vi "Align Window on Parent.vi"(8 "error in (no error)":errorcluster, 10 "Parent VI":refnum<vi>, 11 "VI in":refnum<vi>) -> (0 "error out":errorcluster, 3 "VI out":refnum<vi>)   [LabVIEW 2020]
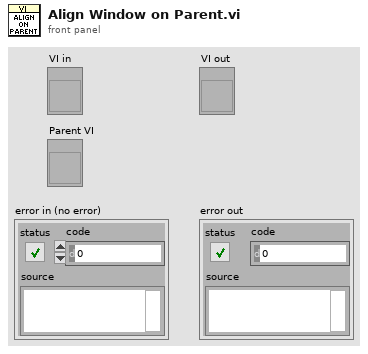
[diagram p1: front panel]
types:
  T1 = typedef "LVRectTypeDef.ctl" = cluster{"Left":i16, "Top":i16, "Right":i16, "Bottom":i16}
  T2 = cluster{i16, "Top":i16, "Right":i16, "Bottom":i16}
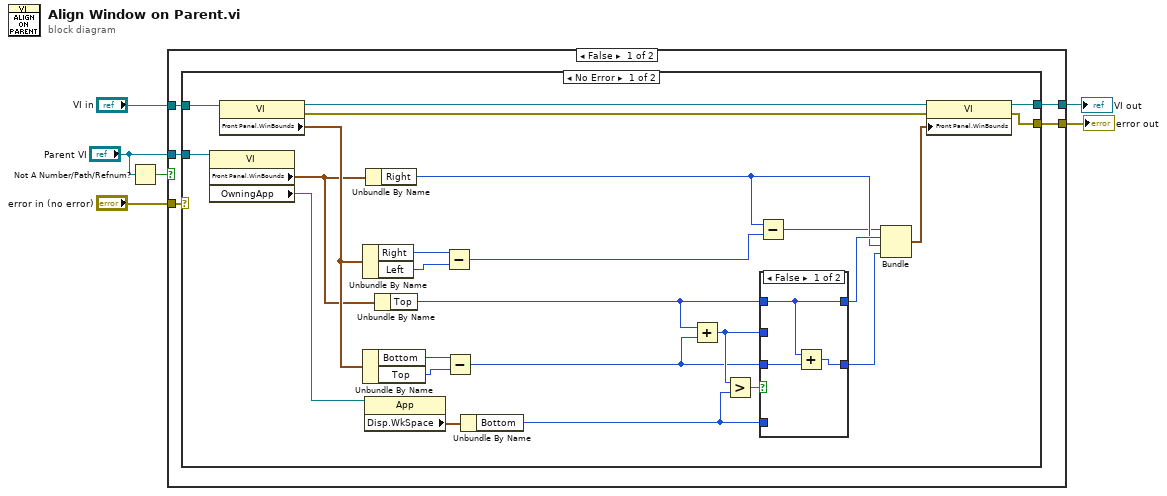
[diagram p0: block diagram]
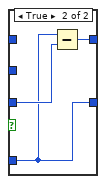
[diagram p2: hidden frame]
diagram:
  n1 = Not A Number/Path/Refnum?(number/path/refnum="Parent VI") -> (NaN/Path/Refnum?=w1:bool)
  n2 = case shown="False" w1 {
    tunnel: [w11 w44] -> w6
    tunnel: [w10 w45] -> w5
    tunnel: "error in (no error)" -> [w9 w45]
    tunnel: "VI in" -> [w8 w44]
    tunnel: "Parent VI" -> [w7 _]
    frame False {
      n3 = case shown="No Error" w9 {
        tunnel: w8 -> [w36 w43]
        tunnel: [w32 _] -> w10
        tunnel: [w33 w43] -> w11
        tunnel: w7 -> [w26 _]
        frame No Error {
          n4 = property class="VI"(reference=w26) -> ("Front Panel.WinBounds"=w25:T1, "OwningApp"=w24:refnum<vi>)  [unwired: 1 in, 2 out]
          n5 = property class="VI"(reference=w36) -> (reference out=w34:refnum<vi>, error out=w35:errorcluster, "Front Panel.WinBounds"=w27:T1)  [unwired: 1 in]
          n6 = Unbundle By Name(w27) -> ("Right"=w31:i16, "Left"=w30:i16)
          n7 = Unbundle By Name(w27) -> ("Bottom"=w29:i16, "Top"=w28:i16)
          n8 = property class="App"(reference=w24) -> ("Disp.WkSpace"=w23:T1)  [unwired: 1 in, 2 out]
          n9 = Unbundle By Name(w25) -> ("Right"=w14:i16)
          n10 = Unbundle By Name(w25) -> ("Top"=w16:i16)
          n11 = Subtract(x=w31, y=w30) -> (x-y=w13:i16)
          n12 = Subtract(x=w29, y=w28) -> (x-y=w17:i16)
          n13 = Unbundle By Name(w23) -> ("Bottom"=w21:i16)
          n14 = Add(x=w16, y=w17) -> (x+y=w20:i16)
          n15 = Greater?(x=w20, y=w21) -> (0:w22:bool)
          n16 = Subtract(x=w14, y=w13) -> (x-y=w12:i16)
          n17 = case shown="False" w22 {
            tunnel: w21 -> [_ w40]
            tunnel: w20 -> [_ _]
            tunnel: w16 -> [w38 _]
            tunnel: [w37 w40] -> w19
            tunnel: [w38 w42] -> w18
            tunnel: w17 -> [w39 w41]
            frame False {
              n18 = Add(x=w38, y=w39) -> (x+y=w37:i16)
            }
            frame True {
              n19 = Subtract(x=w40, y=w41) -> (x-y=w42:i16)
            }
          }
          n20 = Bundle(w12, "Top"=w18, "Right"=w14, "Bottom"=w19) -> (w15:T2)  [unwired: 1 in]
          n21 = property class="VI"(reference=w34, error in=w35, "Front Panel.WinBounds"=w15) -> (reference out=w33:refnum<vi>, error out=w32:errorcluster)
        }
        frame Error {
        }
      }
    }
    frame True {
    }
  }
  "VI out" <- w6
  "error out" <- w5
